vi "Some Thing.vi"(8 "error in (no error)":errorcluster, 11 "Process in":refnum<class "Process.lvclass">) -> (0 "error out":errorcluster, 3 "Process out":refnum<class "Process.lvclass">)   [LabVIEW 2021, in "Process.lvlib" / "Process.lvclass"]
uses:
  Process.lvclass
  AAM/AAM/Self Actor/Self Actor.lvclass
  AAM/AAM/Msg/Msg.lvclass
  Process.lvclass/Process.ctl
  AAM/AAM/Self Actor/Nest Msg Send.vi
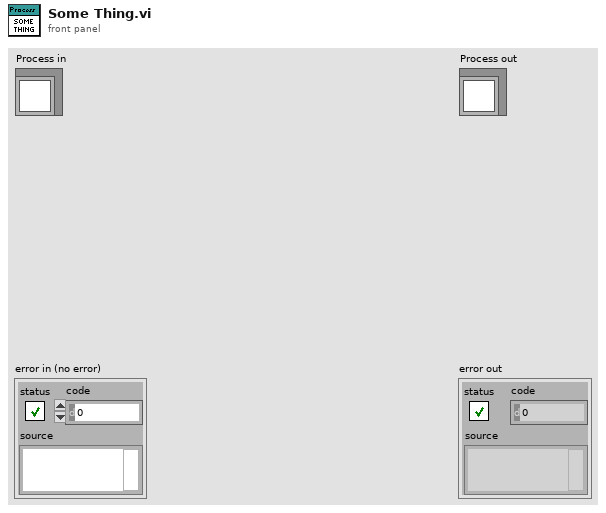
[diagram p1: front panel]
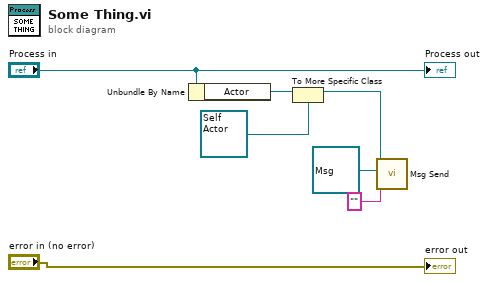
[diagram p0: block diagram]
diagram:
  n1 = Unbundle By Name("Process in") -> ("Actor"=w5:refnum<class "Actor.lvclass">)
  n2 = To More Specific Class(target class=refnum<class "Self Actor.lvclass"> refnum ("AAM.lvlib:Self Actor.lvclass"), reference=w5) -> (specific class reference=w4:refnum<class "Self Actor.lvclass">)  [unwired: 1 in, 1 out]
  n3 = call-poly "Msg Send.vi"("Alias"="", "Msg"=refnum<class "Msg.lvclass"> refnum, "Self Actor in"=w4) -> ()  [unwired: 8 in, 1 out]
  "error out" <- "error in (no error)"
  "Process out" <- "Process in"
